vi "WriteKML.vi"(0 "Latitude":string, 2 "Longitude":string) -> (6 "Path":string)   [LabVIEW 2015]
panel:
  out "error out":errorcluster
  in  "error in":errorcluster
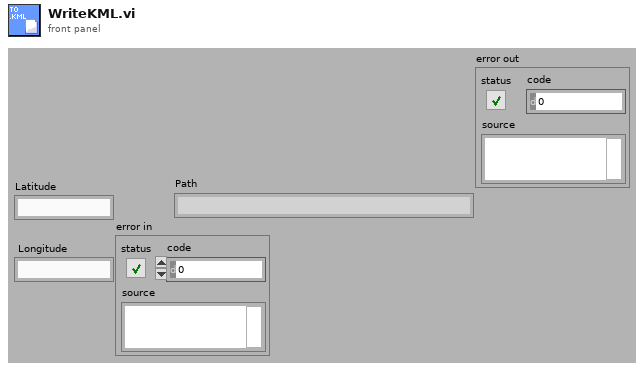
[diagram p1: front panel]
types:
  T1 = enum16{"open", "replace", "create", "open or create", "replace or create", "replace or create with confirmation"}
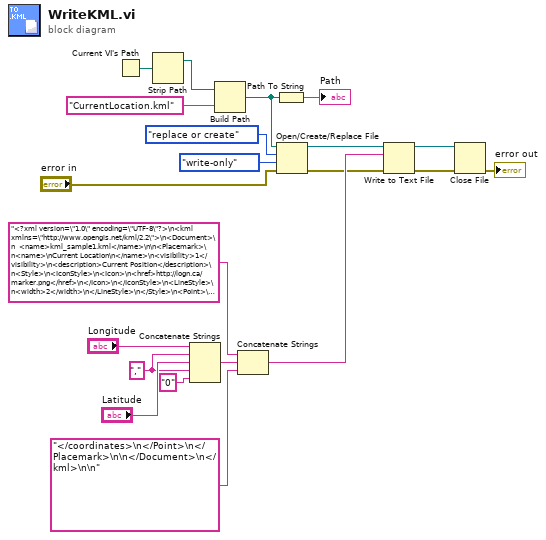
[diagram p0: block diagram]
diagram:
  w16 = ","
  n1 = Current VI's Path() -> (path=w9:path)
  n2 = Strip Path(path=w9) -> (stripped path=w8:path)  [unwired: 1 out]
  n3 = Concatenate Strings("Longitude", w16, "Latitude", w16, "0" ("string")) -> (w17:string)
  n4 = Build Path(base path=w8, name or relative path="CurrentLocation.kml") -> (appended path=w6:path)
  n5 = Concatenate Strings("<?xml version=\"1.0\" encoding=\"UTF-8\"?>\n<kml xmlns=\"http://www.opengis.net/kml/2.2\">\n<Document>\n  <name>kml_sample1.kml</name>\n\n<Placemark>\n<name>\nCurrent Location\n</name>\n<visibility>1</visibility>\n<description>Current Position</description>\n<Style>\n<IconStyle>\n<Icon>\n<href>http://logn.ca/marker.png</href>\n</Icon>\n</IconStyle>\n<LineStyle>\n<width>2</width>\n</LineStyle>\n</Style>\n<Point>\n<extrude>1</extrude>\n<altitudeMode>relativeToGround</altitudeMode>\n<coordinates>", w17, "</coordinates>\n</Point>\n</Placemark>\n\n</Document>\n</kml>\n\n") -> (w14:string)
  n6 = Path To String(path=w6) -> (string=→"Path":string)
  n7 = Open/Create/Replace File(file path (use dialog)=w6, error in="error in", operation (0:open)=T1."replace or create", access (0:read/write)=enum16{"read/write", "read-only", "write-only"}."write-only") -> (refnum out=w13:refnum<file>, error out=w4:errorcluster)  [unwired: 3 out]
  n8 = Write to Text File(file (use dialog)=w13, text=w14, error in=w4) -> (refnum out=w15:refnum<file>, error out=w3:errorcluster)  [unwired: 2 out]
  n9 = Close File(refnum=w15, error in=w3) -> (error out=→"error out":errorcluster)  [unwired: 1 out]
